vi "check_amp.vi"() -> ()   [LabVIEW 2013]
panel:
  out "status 3":bool
  out "status 2":bool
  out "status":bool
  out "current, A":dbl
  out "voltage, V":dbl
  in  "delay before read (ms)":u32=500
  in  "Amp PS address":refnum<visa-resource-name>
  in  "exit":bool
  in  "ps_set":bool
  in  "ps_off":bool
  in  "ps_on":bool
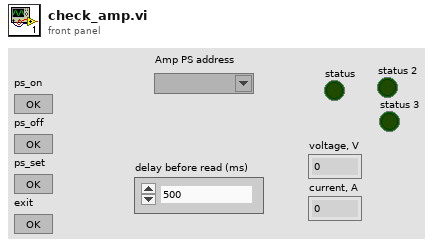
[diagram p1: front panel]
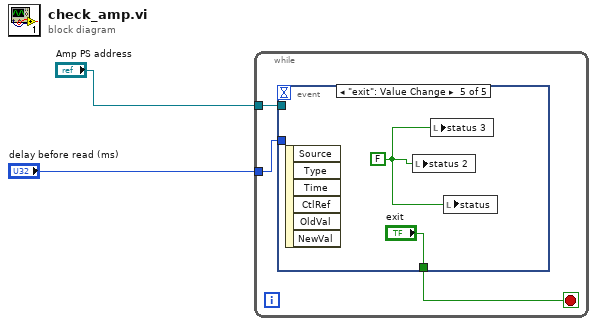
[diagram p0: block diagram]
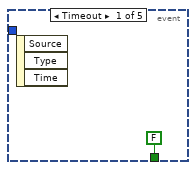
[diagram p2: hidden frame]
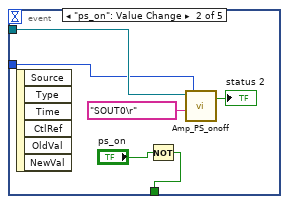
[diagram p3: hidden frame]
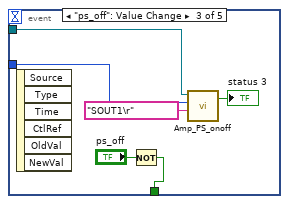
[diagram p4: hidden frame]
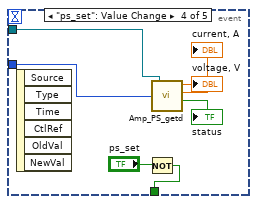
[diagram p5: hidden frame]
diagram:
  n1 = while {
    tunnel: "Amp PS address" -> [w4]
    tunnel: "delay before read (ms)" -> [w3]
    stop <- w5 stop-if-true
    n2 = event shown="[4] \"exit\": Value Change" {
      selector: _ -> [_ _ _ _ _]
      dyn-events: _ -> [_ _ _ _ _]
      timeout: _ -> [_ _ _ _ _]
      tunnel: [FALSE ("exit") w7 w14 w19 "exit"] -> w5
      tunnel: w4 -> [_ w12 w18 w25 _]
      tunnel: w3 -> [_ w11 w17 w24 _]
      event Timeout {
        n3 = event-data() -> ()  [unwired: 1 in, 3 out]
      }
      event "ps_on": Value Change {
        n4 = event-data() -> ()  [unwired: 1 in, 6 out]
        n5 = Not(x="ps_on") -> (.not. x?=w7:bool)
        n6 = call "Amp_PS_onoff.vi"("On/Off Control"="SOUT0\r", "delay before read (ms)"=w11, "Amp PS address"=w12) -> ("status"=→"status 2":bool)  [unwired: 1 in, 1 out]
      }
      event "ps_off": Value Change {
        n7 = event-data() -> ()  [unwired: 1 in, 6 out]
        n8 = Not(x="ps_off") -> (.not. x?=w14:bool)
        n9 = call "Amp_PS_onoff.vi"("On/Off Control"="SOUT1\r", "delay before read (ms)"=w17, "Amp PS address"=w18) -> ("status"=→"status 3":bool)  [unwired: 1 in, 1 out]
      }
      event "ps_set": Value Change {
        n10 = event-data() -> ()  [unwired: 1 in, 6 out]
        n11 = Not(x="ps_set") -> (.not. x?=w19:bool)
        n12 = call "Amp_PS_getd.vi"("Amp PS address"=w25, "delay before read (ms)"=w24) -> ("voltage, V"=→"voltage, V":dbl, "current, A"=→"current, A":dbl, "status"=→"status":bool)  [unwired: 1 in, 2 out]
      }
      event "exit": Value Change {
        w26 = FALSE
        n13 = event-data() -> ()  [unwired: 1 in, 6 out]
        n14 = local write "status 2"(w26) -> ()
        n15 = local write "status 3"(w26) -> ()
        n16 = local write "status"(w26) -> ()
      }
    }
  }
